vi "dfd_Error Handlers.vi"   [LabVIEW 2017, in "NI_DigFilterLicensed.lvlib"]
uses:
  <vilib>/addons/Digital Filter Design/NI_DigFilterLicensed.lvlib
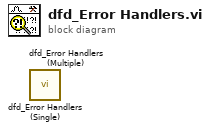
[diagram p0: block diagram]
diagram:
  n1 = call <vilib>:"dfd_Error Handlers (Single).vi"() -> ()  [unwired: 11 in, 1 out]
  n2 = call <vilib>:"dfd_Error Handlers (Multiple).vi"() -> ()  [unwired: 11 in, 1 out]
